vi "Version Cluster to String.vi"(11 "version":T1) -> (3 "version string":string)   [LabVIEW 2017, in "DSF System Explorer.lvlib"]
uses:
  DSF System Explorer.lvlib
  DSF Core.lvlibp/Typedefs/DSF Version Info.ctl
  DSF Core.lvlibp
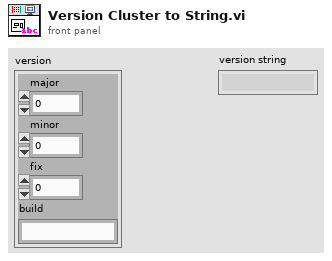
[diagram p1: front panel]
types:
  T1 = typedef "DSF Core.lvlibp/DSF Version Info.ctl" = cluster{"major":u32, "minor":u32, "fix":u32, "build":string}
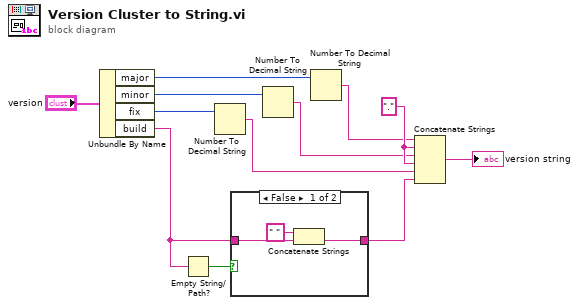
[diagram p0: block diagram]
diagram:
  w8 = "."
  n1 = Unbundle By Name("version") -> ("major"=w11:u32, "minor"=w10:u32, "fix"=w9:u32, "build"=w4:string)
  n2 = Empty String/Path?(string/path=w4) -> (empty?=w3:bool)
  n3 = Number To Decimal String(number=w9) -> (decimal integer string=w5:string)  [unwired: 1 in]
  n4 = case shown="False" w3 {
    tunnel: w4 -> [w14 w16]
    tunnel: [w13 w16] -> w2
    frame False {
      n5 = Concatenate Strings(" " ("string"), w14) -> (w13:string)
    }
    frame True {
    }
  }
  n6 = Number To Decimal String(number=w10) -> (decimal integer string=w6:string)  [unwired: 1 in]
  n7 = Number To Decimal String(number=w11) -> (decimal integer string=w7:string)  [unwired: 1 in]
  n8 = Concatenate Strings(w7, w8, w6, w8, w5, w2) -> (→"version string":string)
